vi "GetString.vi"(7 "group":string, 8 "error in (no error)":errorcluster, 10 "param":string, 11 "ConfigClass_IN":refnum<class "ConfigClass.lvclass">) -> (0 "error out":errorcluster, 2 "string_out":string, 3 "ConfigClass_OUT":refnum<class "ConfigClass.lvclass">)   [LabVIEW 2019, in "ConfigClass.lvlib" / "ConfigClass.lvclass"]
uses:
  ConfigClass.lvclass
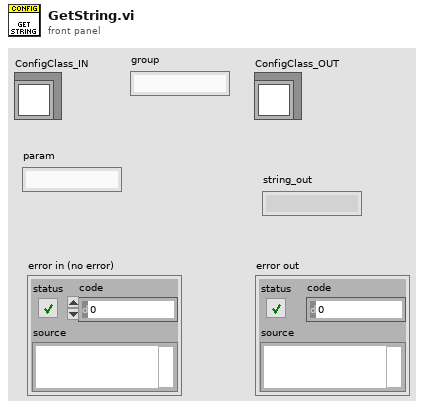
[diagram p1: front panel]
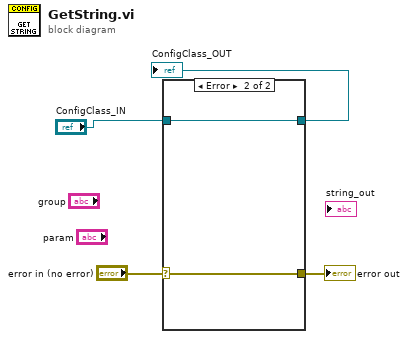
[diagram p0: block diagram]
diagram:
  n1 = case shown="Error" "error in (no error)" {
    selector: "error in (no error)" -> [w6 w7]
    tunnel: [w6 w7] -> w3
    tunnel: [w5 w8] -> w2
    tunnel: "ConfigClass_IN" -> [w5 w8]
    frame No Error {
    }
    frame Error {
    }
  }
  "error out" <- w3
  "ConfigClass_OUT" <- w2
